vi "Load_NN_Model_Weights.vi"() -> ()   [LabVIEW 2023]
uses:
  <vilib>/Utility/file.llb/Read Delimited Spreadsheet (DBL).vi
  NN_model_params.vi
panel:
  out "full_paths":path[](array[path])
  out "Array":bool[](array[boolean])
  out "filenames":string[](array[string])
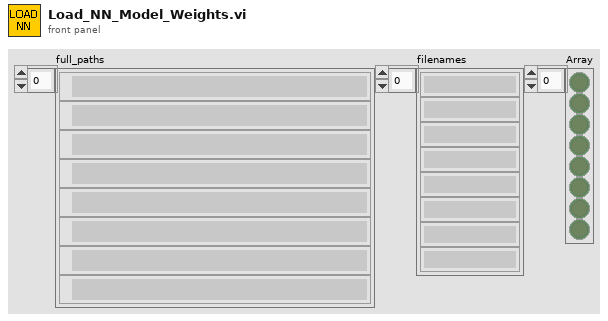
[diagram p1: front panel]
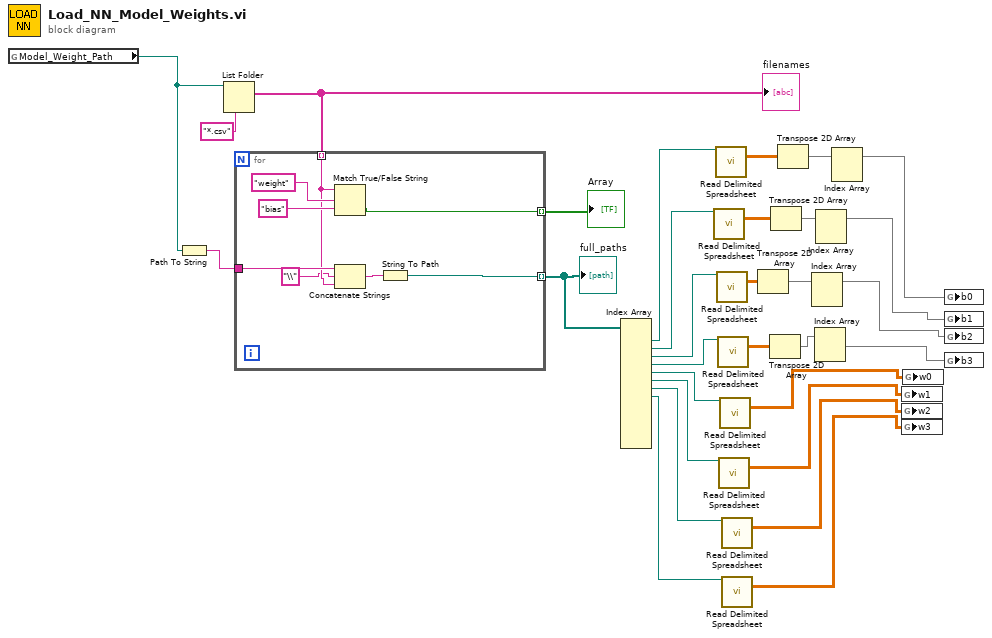
[diagram p0: block diagram]
diagram:
  n1 = global read "NN_model_params.vi" "Model_Weight_Path"() -> (w1:path)
  n2 = Path To String(path=w1) -> (string=w27:string)
  n3 = List Folder(path=w1, pattern="*.csv") -> (filenames=w29:string[])  [unwired: 2 in, 3 out]
  "filenames" <- w29
  n4 = for {
    tunnel: w29 -> [w32] mode=indexing
    tunnel: [w36] -> w28 mode=indexing
    tunnel: w27 -> [w35]
    tunnel: [w33] -> w25 mode=indexing
    n5 = Match True/False String(2:"bias" ("false string"), 3:"weight" ("true string"), 4:w32) -> (0:w36:bool)  [unwired: 1 out]
    n6 = Concatenate Strings(w35, "\\" ("string"), w32) -> (w34:string)
    n7 = String To Path(string=w34) -> (path=w33:path)
  }
  "Array" <- w28
  "full_paths" <- w25
  n8 = Index Array(array=w25) -> (element #1=w26:path, element #2=w24:path, element #3=w23:path, element #4=w22:path, element #5=w21:path, element #6=w20:path, element #7=w19:path, element #8=w18:path)  [unwired: 14 in, 6 out]
  n9 = call-poly <vilib>:"Read Delimited Spreadsheet.vi"("file path (dialog if empty)"=w24) -> ("all rows"=w16:dbl[][])  [unwired: 9 in, 5 out]
  n10 = call-poly <vilib>:"Read Delimited Spreadsheet.vi"("file path (dialog if empty)"=w26) -> ("all rows"=w17:dbl[][])  [unwired: 9 in, 5 out]
  n11 = call-poly <vilib>:"Read Delimited Spreadsheet.vi"("file path (dialog if empty)"=w23) -> ("all rows"=w15:dbl[][])  [unwired: 9 in, 5 out]
  n12 = call-poly <vilib>:"Read Delimited Spreadsheet.vi"("file path (dialog if empty)"=w22) -> ("all rows"=w14:dbl[][])  [unwired: 9 in, 5 out]
  n13 = call-poly <vilib>:"Read Delimited Spreadsheet.vi"("file path (dialog if empty)"=w20) -> ("all rows"=w4:dbl[][])  [unwired: 9 in, 5 out]
  n14 = call-poly <vilib>:"Read Delimited Spreadsheet.vi"("file path (dialog if empty)"=w21) -> ("all rows"=w5:dbl[][])  [unwired: 9 in, 5 out]
  n15 = call-poly <vilib>:"Read Delimited Spreadsheet.vi"("file path (dialog if empty)"=w19) -> ("all rows"=w3:dbl[][])  [unwired: 9 in, 5 out]
  n16 = call-poly <vilib>:"Read Delimited Spreadsheet.vi"("file path (dialog if empty)"=w18) -> ("all rows"=w2:dbl[][])  [unwired: 9 in, 5 out]
  n17 = Transpose 2D Array(2D array=w15) -> (transposed array=w11:dbl[][])
  n18 = Transpose 2D Array(2D array=w14) -> (transposed array=w10:dbl[][])
  n19 = Transpose 2D Array(2D array=w16) -> (transposed array=w12:dbl[][])
  n20 = Transpose 2D Array(2D array=w17) -> (transposed array=w13:dbl[][])
  n21 = Index Array(array=w11) -> (element=w7:dbl[])  [unwired: 2 in]
  n22 = Index Array(array=w10) -> (element=w6:dbl[])  [unwired: 2 in]
  n23 = Index Array(array=w12) -> (element=w8:dbl[])  [unwired: 2 in]
  n24 = Index Array(array=w13) -> (element=w9:dbl[])  [unwired: 2 in]
  n25 = global write "NN_model_params.vi" "w1"(w4) -> ()
  n26 = global write "NN_model_params.vi" "w2"(w3) -> ()
  n27 = global write "NN_model_params.vi" "w3"(w2) -> ()
  n28 = global write "NN_model_params.vi" "w0"(w5) -> ()
  n29 = global write "NN_model_params.vi" "b0"(w9) -> ()
  n30 = global write "NN_model_params.vi" "b1"(w8) -> ()
  n31 = global write "NN_model_params.vi" "b2"(w7) -> ()
  n32 = global write "NN_model_params.vi" "b3"(w6) -> ()
